vi "Buffer.vi"(9 "MaxSize":i32, 11 "InputData":dbl) -> (3 "Buffer":ext[](array[numeric]))   [LabVIEW 2019]
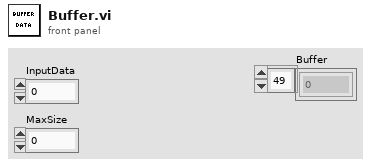
[diagram p1: front panel]
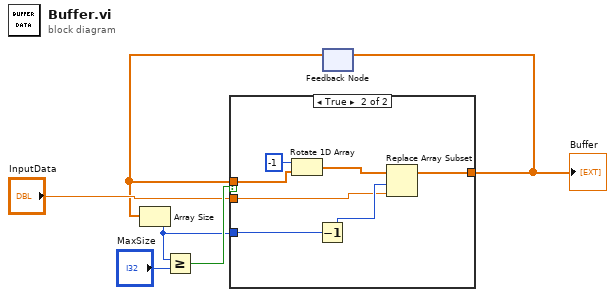
[diagram p0: block diagram]
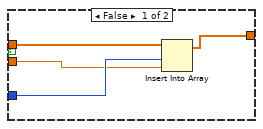
[diagram p2: hidden frame]
diagram:
  n1 = feedback #1() -> (w1:dbl[])  [unwired: 1 in]
  n2 = Array Size(array=w1) -> (size(s)=w3:i32)
  n3 = Greater Or Equal?(x=w3, y="MaxSize") -> (x >= y?=w5:bool)
  n4 = case shown="True" w5 {
    tunnel: w1 -> [w8 w16]
    tunnel: "InputData" -> [w9 w12]
    tunnel: w3 -> [w10 w15]
    tunnel: [w7 w11] -> w2
    frame False {
      n5 = Insert Into Array(array=w8, index=w10, new element=w9) -> (w7:dbl[])
    }
    frame True {
      n6 = Rotate 1D Array(1:w16, 2:-1 ("n")) -> (0:w13:dbl[])
      n7 = Decrement(x=w15) -> (x-1=w14:i32)
      n8 = Replace Array Subset(array=w13, new element=w12, index=w14) -> (w11:dbl[])
    }
  }
  "Buffer" <- w2
  n9 = feedback-in #1(w2) -> ()
